vi "Condition Conpane Map.vi"(8 "error in":errorcluster, 9 "Ref.Name VI (Interface)":refnum<vi>, 10 "Control FP Order":i32[](array[numeric])) -> (0 "error out":errorcluster, 2 "Conpane Map":T1(c390))   [LabVIEW 2025, in "_Msg Rescript.lvlib" / "_Msg Rescript.lvclass"]
uses:
  _Msg Rescript.lvclass
  _Msg Rescript.lvclass/_Msg Rescript.ctl
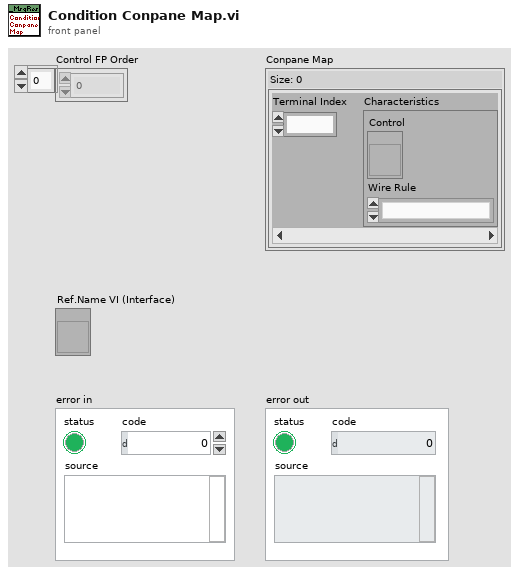
[diagram p1: front panel]
types:
  T1 = map{i32, cluster{"Control":refnum<vi>, "Wire Rule":enum16{"Invalid Wire Rule", "Required", "Recommended", "Optional", "Dynamic Dispatch"}}}
  T2 = enum16{"Invalid Wire Rule", "Required", "Recommended", "Optional", "Dynamic Dispatch"}[]
  T3 = cluster{"Control":refnum<vi>, "Wire Rule":enum16{"Invalid Wire Rule", "Required", "Recommended", "Optional", "Dynamic Dispatch"}}
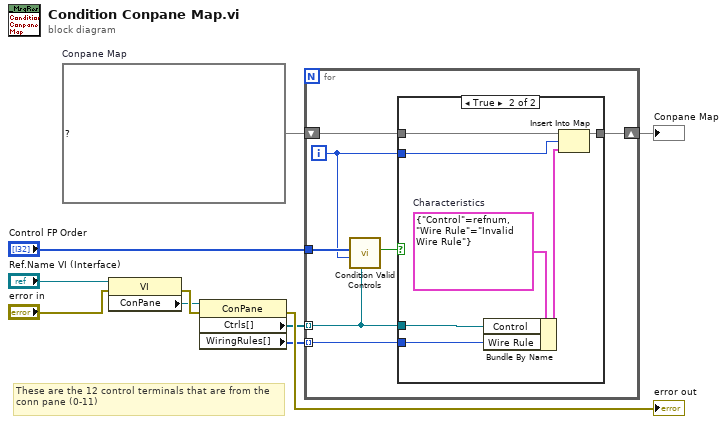
[diagram p0: block diagram]
diagram:
  w7 = T1 {}  # Conpane Map
  # "These are the 12 control terminals that are from the conn pane (0-11)"
  n1 = property class="VI"(reference="Ref.Name VI (Interface)", error in="error in") -> (error out=w9:errorcluster, "ConPane"=w8:refnum<vi>)  [unwired: 1 out]
  n2 = property class="ConPane"(reference=w8, error in=w9) -> (error out=→"error out":errorcluster, "Ctrls[]"=w1:refnum<vi>[], "WiringRules[]"=w6:T2)  [unwired: 1 out]
  n3 = for {
    tunnel: "Control FP Order" -> [w13]
    shift-right: [w17] -> w3
    shift-left: w7 -> [w16]
    tunnel: w1 -> [w11] mode=indexing
    tunnel: w6 -> [w15] mode=indexing
    i -> [w12]
    n4 = call "Condition Valid Controls.vi"("Ctl Refnum"=w11, "Terminal Index"=w12, "Control Terminals"=w13) -> ("Valid"=w14:bool)  [unwired: 8 in]
    n5 = case shown="True" w14 {
      tunnel: [w18 w25] -> w17
      tunnel: w16 -> [w18 w24]
      tunnel: w15 -> [_ w23]
      tunnel: w12 -> [_ w22]
      tunnel: w11 -> [_ w21]
      frame False {
      }
      frame True {
        w20 = T3 {"Control"=refnum, "Wire Rule"=enum."Invalid Wire Rule"}  # Characteristics
        n6 = Bundle By Name(cluster=w20, "Control"=w21, "Wire Rule"=w23) -> (w19:T3)
        n7 = Insert Into Map(map in=w24, key=w22, value=w19) -> (map out=w25:T1)  [unwired: 2 out]
      }
    }
  }
  "Conpane Map" <- w3
